vi "BrowseCLI.vi"() -> ()   [LabVIEW 2012]
panel:
  out "Strings":string[](array[string])
  out "Plot":cluster{"Plot":cluster{"X":dbl, "Y":dbl}[]}[](graph)
  out "Commands":T1(array[cluster])
  in  "Browse For CLI":path
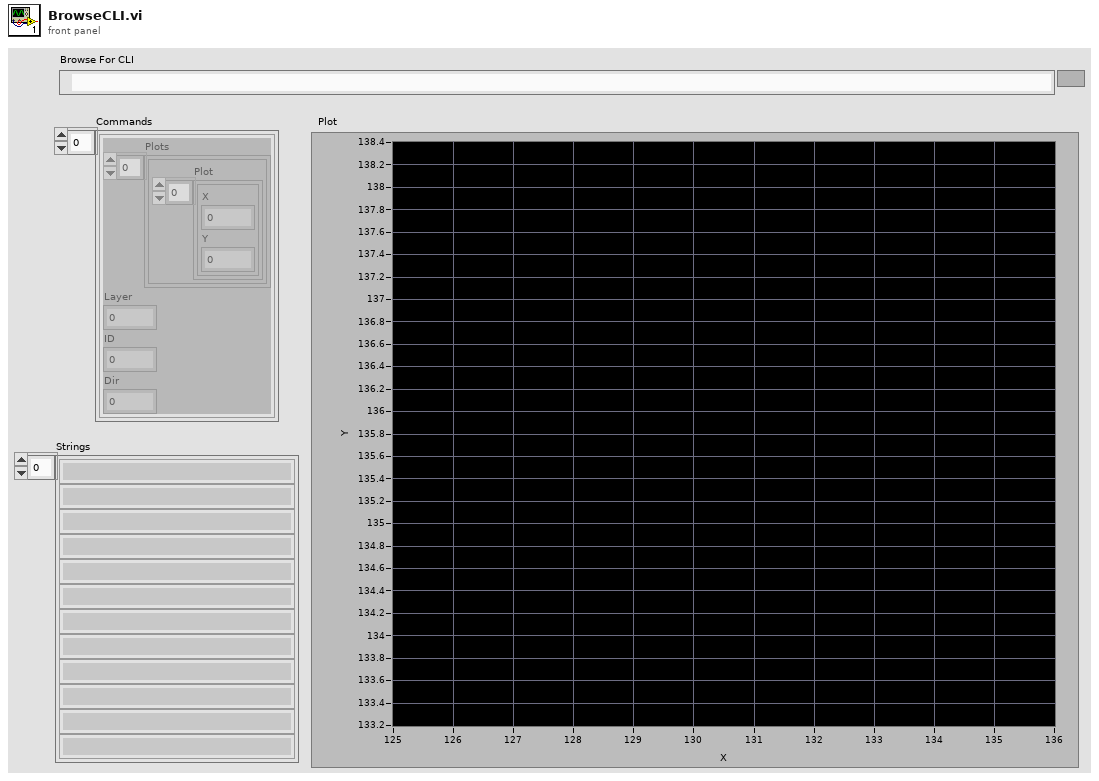
[diagram p1: front panel]
types:
  T1 = cluster{"Plots":cluster{"Plot":cluster{"X":dbl, "Y":dbl}[]}[], "Layer":dbl, "ID":dbl, "Dir":dbl}[]
  T2 = cluster{"Plots":cluster{"Plot":cluster{"X":dbl, "Y":dbl}[]}[], "Layer":dbl, "ID":dbl, "Dir":dbl}
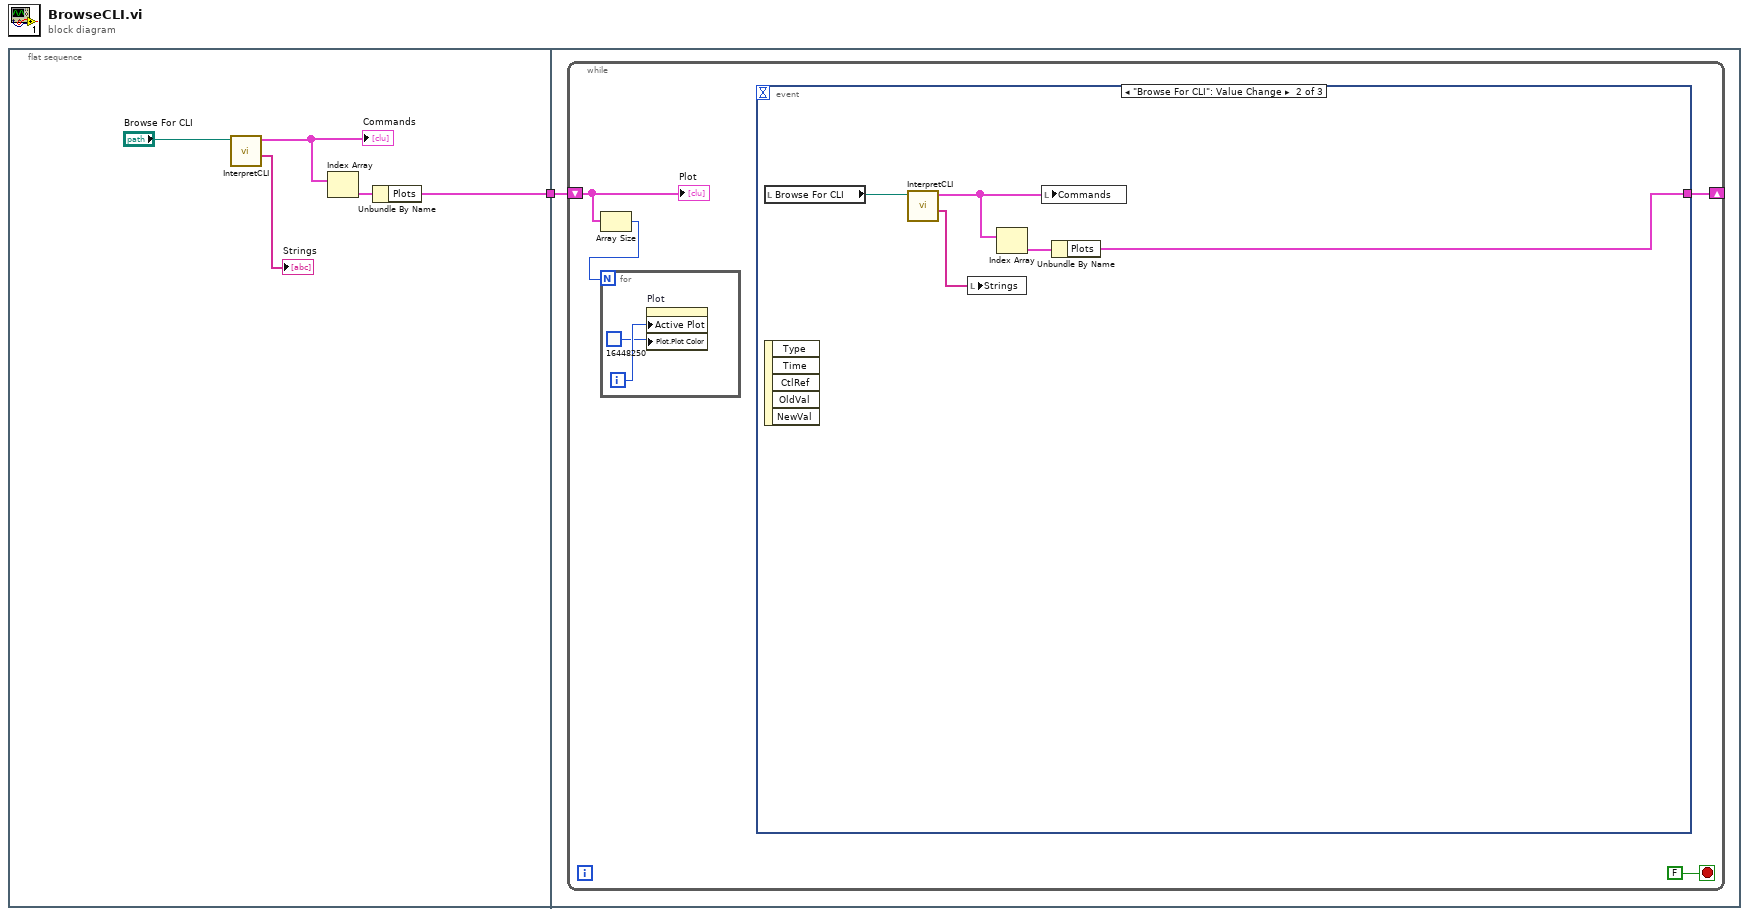
[diagram p0: block diagram]
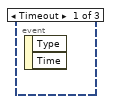
[diagram p2: hidden frame]
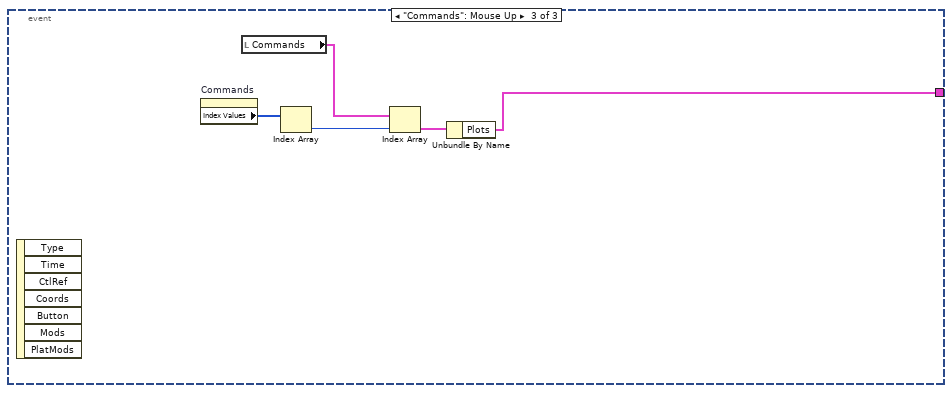
[diagram p3: hidden frame]
diagram:
  n1 = flat-sequence {
    tunnel: [w4] -> w1
    tunnel: w1 -> [w7]
    frame #0 {
      n2 = call "InterpretCLI.vi"("Path"="Browse For CLI") -> ("Strings"=→"Strings":string[], "Commands"=w6:T1)  [unwired: 8 in, 1 out]
      "Commands" <- w6
      n3 = Index Array(array=w6) -> (element=w5:T2)  [unwired: 1 in]
      n4 = Unbundle By Name(w5) -> ("Plots"=w4:cluster{"Plot":cluster{"X":dbl, "Y":dbl}[]}[])
    }
    frame #1 {
      n5 = while {
        shift-right: [w10] -> _
        shift-left: w7 -> [w9]
        stop <- FALSE stop-if-true
        n6 = Array Size(array=w9) -> (size(s)=w8:i32)
        n7 = for {
          N: w8 -> [_]
          i -> [w13]
          n8 = property on="Plot" class="XYGraph (strict)"("Active Plot"=w13, "Plot.Plot Color"=u32 16448250) -> ()  [unwired: 2 in, 2 out]
        }
        n9 = event shown="[1] \"Browse For CLI\": Value Change" {
          selector: _ -> [_ _ _]
          dyn-events: _ -> [_ _ _]
          timeout: _ -> [_ _ _]
          tunnel: [_ w15 w19] -> w10
          event Timeout {
            n10 = event-data() -> ()  [unwired: 1 in, 2 out]
          }
          event "Browse For CLI": Value Change {
            n11 = local read "Browse For CLI"() -> (w18:path)
            n12 = event-data() -> ()  [unwired: 1 in, 5 out]
            n13 = call "InterpretCLI.vi"("Path"=w18) -> ("Strings"=w14:string[], "Commands"=w17:T1)  [unwired: 8 in, 1 out]
            n14 = local write "Strings"(w14) -> ()
            n15 = Index Array(array=w17) -> (element=w16:T2)  [unwired: 1 in]
            n16 = local write "Commands"(w17) -> ()
            n17 = Unbundle By Name(w16) -> ("Plots"=w15:cluster{"Plot":cluster{"X":dbl, "Y":dbl}[]}[])
          }
          event "Commands": Mouse Up {
            n18 = event-data() -> ()  [unwired: 1 in, 7 out]
            n19 = property on="Commands" class="Arr (strict)"() -> ("Index Values"=w23:u32[])  [unwired: 2 in, 2 out]
            n20 = local read "Commands"() -> (w21:T1)
            n21 = Index Array(array=w23) -> (element=w20:u32)  [unwired: 1 in]
            n22 = Index Array(array=w21, index=w20) -> (element=w22:T2)
            n23 = Unbundle By Name(w22) -> ("Plots"=w19:cluster{"Plot":cluster{"X":dbl, "Y":dbl}[]}[])
          }
        }
        "Plot" <- w9
      }
    }
  }
